vi "Wave1D_Insert Sol.vi"(9 "time step":i32, 10 "Wave1D Data":T1 {"BC"."End X"."type" items=["Dirichlet", "Neumann"]; "BC"."Start X"."type" items=["Dirichlet", "Neumann"]}, 11 "U(t, x) In":dbl[][](array[numeric])) -> (3 "U(t, x) Out":dbl[][](array[numeric]))   [LabVIEW 2020, in "NI_PDE.lvlib"]
uses:
  <vilib>/gmath/NI_PDE.lvlib
  <vilib>/gmath/pde.llb/Wave1D/Wave1D_Data.ctl
  <vilib>/gmath/pde.llb/Common/PDE_BC Type.ctl
  <vilib>/Analysis/Matrix/Datatypes/RealMatrix.ctl
  <vilib>/Analysis/Matrix/NI_Matrix.lvlib
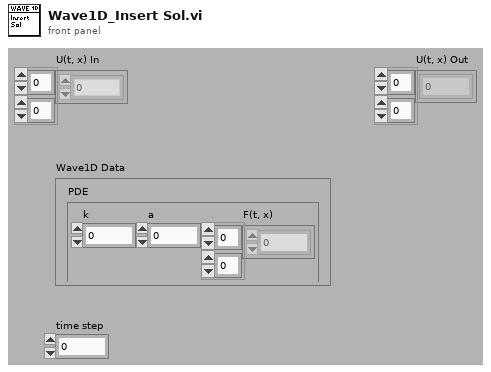
[diagram p1: front panel]
types:
  T1 = typedef "NI_PDE.lvlib/Wave1D_Data.ctl" = cluster{"PDE":cluster{"k":dbl, "a":dbl, "F(t, x)":dbl[][]}, "Domain":cluster{"t":cluster{"initial t":dbl, "final t":dbl, "# of t-points":i32}, "x":cluster{"start x":dbl, "end x":dbl, "# of x-points":i32}, "delta":cluster{"delta t":dbl, "delta x":dbl}}, "BC":cluster{"Start X":cluster{"type":T2, "Value":dbl[]}, "End X":cluster{"type":T2, "Value":dbl[]}}, "IC":cluster{"Value":dbl[], "Derivative":dbl[]}, "A":cluster{"Sub Diag":dbl[], "Diag":dbl[], "Super Diag":dbl[], "A":T3}, "LU of A":cluster{"L":dbl[], "U":cluster{"Diag":dbl[], "Super Diag":dbl[], "2nd Super Diag":dbl[]}, "Pivot":i32[]}, "State":cluster{"U":dbl[], "AU":dbl[], "Old AU":dbl[], "start index":i32, "length":i32}}
  T2 = typedef "NI_PDE.lvlib/PDE_BC Type.ctl" = i32
  T3 = typedef "NI_Matrix.lvlib/RealMatrix.ctl" = dbl[][]
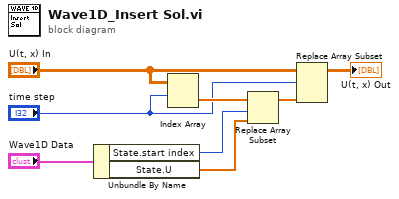
[diagram p0: block diagram]
diagram:
  n1 = Unbundle By Name("Wave1D Data") -> ("State.start index"=w4:i32, "State.U"=w3:dbl[])
  n2 = Index Array(array="U(t, x) In", index (row)="time step") -> (element=w5:dbl[])  [unwired: 1 in]
  n3 = Replace Array Subset(array=w5, new element=w3, index=w4) -> (w2:dbl[])
  n4 = Replace Array Subset(array="U(t, x) In", new element=w2, index (row)="time step") -> (→"U(t, x) Out":dbl[][])  [unwired: 1 in]
